vi "Test Method Result Error Count.vi"(8 "error in (no error)":errorcluster, 11 "Pass Assertion Test In":refnum<class "Method Result Test.lvclass">) -> (0 "error out":errorcluster, 3 "Pass Assertion Test Out":refnum<class "Method Result Test.lvclass">)   [LabVIEW 2020, in "LUnit Tests.lvlib" / "Method Result Test.lvclass"]
uses:
  Method Result Test.lvclass
  C:/Program Files (x86)/National Instruments/LabVIEW 2020/vi.lib/Asteme/LUnit/Test Case.lvclass
  source/Framework/Result Classes/Method Result/Method Result.lvclass/Method Result.ctl
  source/Framework/Result Classes/Assertion Result/Assertion Result.lvclass/Assertion Result.ctl
  <vilib>/Asteme/LUnit/Test Case.lvclass/Test Case.ctl
  <vilib>/Asteme/LUnit/LUnit Assertion Result.lvclass/LUnit Assertion Result.ctl
  <vilib>/Asteme/LUnit/LUnit Test Case Result.lvclass/LUnit Test Case Result.ctl
  <vilib>/Asteme/LUnit/LUnit Method Result.lvclass/LUnit Method Result.ctl
  source/Framework/Result Classes/Method Result/Private/SubVIs/Count Status.vi
  <vilib>/Asteme/LUnit/Palette/Pass.vi
  <vilib>/Asteme/LUnit/Palette/Fail.vi
  <vilib>/Asteme/LUnit/Variant to string.vi
  <vilib>/Asteme/LUnit/Set Assertion Type.vi
  source/Framework/Result Classes/Assertion Result/Public/Read Status.vi
  <vilib>/Asteme/LUnit/Add test result.vi
  <vilib>/Asteme/LUnit/LUnit Write Passed.vi
  <vilib>/Asteme/LUnit/LUnit Write Message.vi
  <vilib>/Asteme/LUnit/LUnit Write Description.vi
  <vilib>/Asteme/LUnit/LUnit Write Assertion Type.vi
  <vilib>/Asteme/LUnit/LUnit Record Assertion Result.vi
  <vilib>/Asteme/LUnit/LUnit Aggregate Assertion Results.vi
  <vilib>/Asteme/LUnit/Assertion Result/LUnit Read Status.vi
  <vilib>/Asteme/LUnit/LUnit Read Message.vi
  <vilib>/Asteme/LUnit/LUnit Read Description.vi
  <vilib>/Asteme/LUnit/Method Result/LUnit Merge Status.vi
  <vilib>/Asteme/LUnit/LUnit Concatenate result strings.vi
  <vilib>/Utility/Data Type/Get Type Information.vi
  <vilib>/Utility/LVClass/Get LV Class Name.vi
  <vilib>/Asteme/LUnit/LUnit Assertion Result.lvclass
  <vilib>/Asteme/LUnit/Test Case.lvclass
  source/Framework/Result Classes/Method Result/Method Result.lvclass
  C:/Users/anton/Documents/GitHub/LUnit/tests/Framework Test/Assertion Test/Method Result Test.lvclass
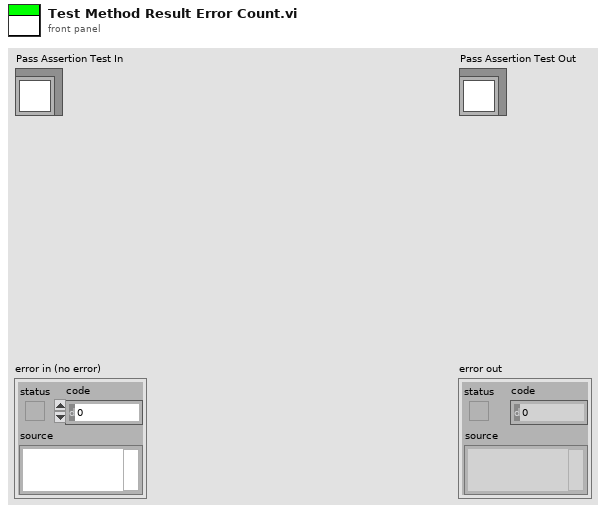
[diagram p1: front panel]
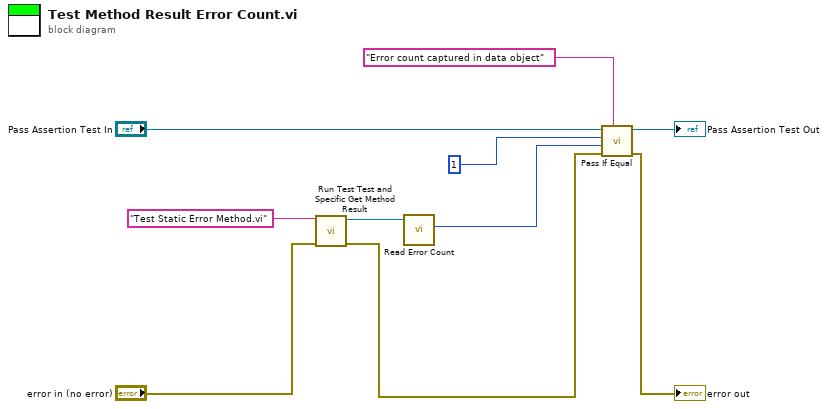
[diagram p0: block diagram]
diagram:
  n1 = call "Run Test Test and Specific Get Method Result.vi"("error in (no error)"="error in (no error)", "Method of Interest"="Test Static Error Method.vi") -> ("error out"=w2:errorcluster, "Method Result out"=w1:refnum<class "Method Result.lvclass">)  [unwired: 8 in]
  n2 = call "Read Error Count.vi"("Method Result In"=w1) -> ("Error count"=w6:i32)  [unwired: 9 in, 1 out]
  n3 = call <vilib>:"Pass If Equal.vi"("Description"="Error count captured in data object", "error in (no error)"=w2, "Actual"=w6, "Expected"=1 ("Assertions count"), "LUnit Test Case In"="Pass Assertion Test In") -> ("error out"=→"error out":errorcluster, "LUnit Test Case Out"=→"Pass Assertion Test Out":refnum<class "Method Result Test.lvclass">)  [unwired: 5 in]
